vi "Write Homed.vi"(8 "error in (no error)":errorcluster, 10 "Homed":T1, 11 "XY Stage Data Class in":refnum<class "XY Stage Data Class.lvclass">) -> (0 "error out":errorcluster, 3 "XY Stage Data Class out":refnum<class "XY Stage Data Class.lvclass">)   [LabVIEW 2022 SP3, in "XY Stage Data Class.lvclass"]
uses:
  XY Stage Data Class.lvclass
  Homed.ctl
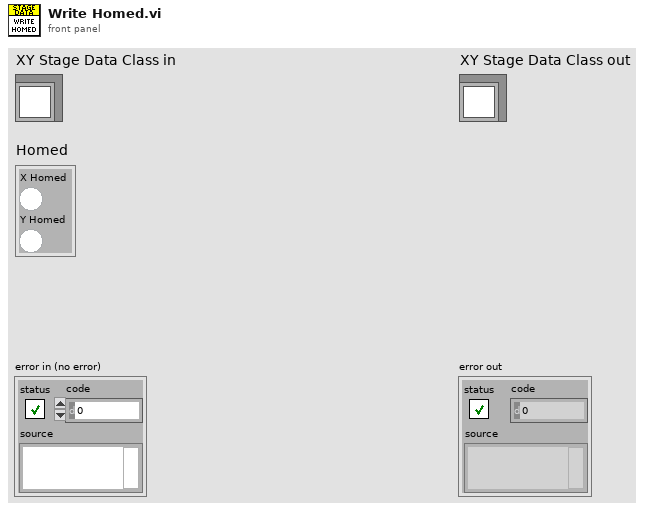
[diagram p1: front panel]
types:
  T1 = typedef "XY Stage Data Class.lvclass/Homed.ctl" = cluster{"X Homed":bool, "Y Homed":bool}
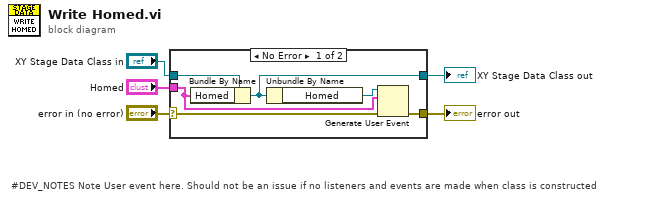
[diagram p0: block diagram]
diagram:
  # "#DEV_NOTES Note User event here. Should not be an issue if no listeners and events are made when class is constructed"
  n1 = case shown="No Error" "error in (no error)" {
    selector: "error in (no error)" -> [w7 w12]
    tunnel: [w6 w12] -> w4
    tunnel: [w10 w13] -> w2
    tunnel: "XY Stage Data Class in" -> [w11 w13]
    tunnel: "Homed" -> [w9 _]
    frame No Error {
      n2 = Bundle By Name(cluster=w11, "Homed"=w9) -> (w10:refnum<class "XY Stage Data Class.lvclass">)
      n3 = Unbundle By Name(w10) -> ("Homed"=w8:refnum<user-event>)
      n4 = Generate User Event(user event=w8, event data cluster=w9, error in=w7) -> (error out=w6:errorcluster)  [unwired: 1 in, 1 out]
    }
    frame Error {
    }
  }
  "error out" <- w4
  "XY Stage Data Class out" <- w2
